vi "Update Parameter Value.vi"(8 "error in (no error)":errorcluster, 9 "Value":dbl format="%#_13g", 10 "Parameter":string, 11 "Async Message in":refnum<class "Async Message.lvclass">) -> (0 "error out":errorcluster, 3 "Async Message out":refnum<class "Async Message.lvclass">)   [LabVIEW 2020, in "BCI-1553 API.lvlib" / "Async Message.lvclass"]
doc: "This method allows a parameter value stored in an Asynchronous Message to be updated."
uses:
  Async Message.lvclass
  Async Message.lvclass/Async Message.ctl
  BCI-1553 API.lvlib
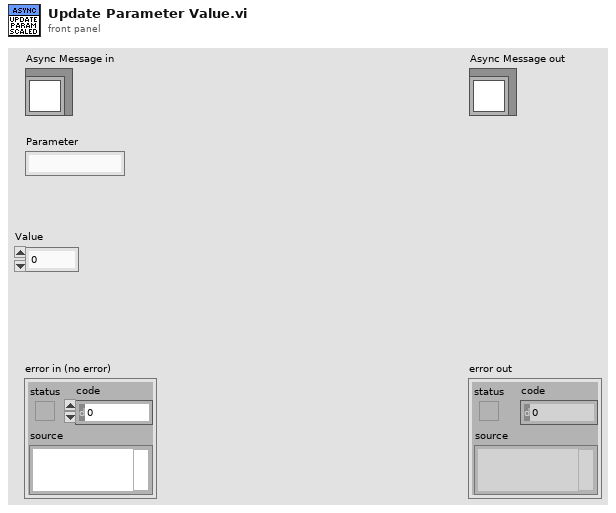
[diagram p1: front panel]
types:
  T1 = typedef "BCI-1553 API.lvlib/Parameter Table Data.ctl" = cluster{"Parameter Name":string, "Base Word":u16, "Address":u16, "Value":u64, "Mask":u16[], "Scaling Info":T2}
  T2 = typedef "BCI-1553 API.lvlib/Scaling Information.ctl" = cluster{"Bit Offset":i32, "Bit Count":i32, "LSB Resolution":dbl, "2's Complement":bool, "Big Endian":bool, "Sign Bit":bool}
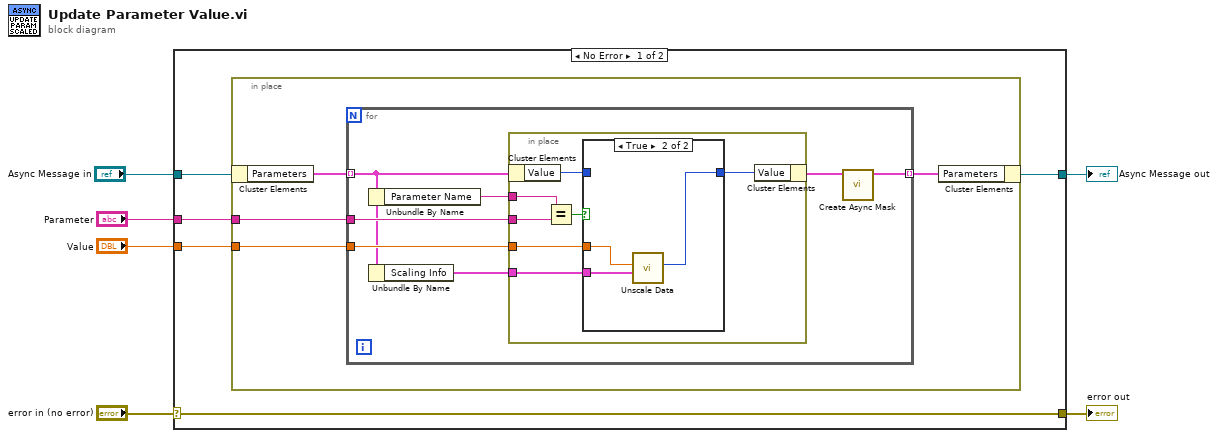
[diagram p0: block diagram]
diagram:
  n1 = case shown="No Error" "error in (no error)" {
    selector: "error in (no error)" -> [w11 w35]
    tunnel: [w11 w35] -> w5
    tunnel: [w7 w34] -> w3
    tunnel: "Async Message in" -> [w8 w34]
    tunnel: "Parameter" -> [w10 _]
    tunnel: "Value" -> [w9 _]
    frame No Error {
      n2 = in-place {
        in-place-border: w10 -> [w15]
        in-place-border: w9 -> [w14]
        n3 = in-place-cluster #1(w8) -> ("Parameters"=w13:T1[])
        n4 = for {
          tunnel: w13 -> [w20] mode=indexing
          tunnel: w15 -> [w22]
          tunnel: w14 -> [w21]
          tunnel: [w16] -> w12 mode=indexing
          n5 = Unbundle By Name(w20) -> ("Parameter Name"=w18:string)
          n6 = Unbundle By Name(w20) -> ("Scaling Info"=w19:T2)
          n7 = in-place {
            in-place-border: w22 -> [w29]
            in-place-border: w21 -> [w25]
            in-place-border: w19 -> [w24]
            in-place-border: w18 -> [w23]
            n8 = in-place-cluster #2(w20) -> ("Value"=w27:u64)
            n9 = Equal?(x=w23, y=w29) -> (x = y?=w28:bool)
            n10 = case shown="True" w28 {
              tunnel: w27 -> [w30 _]
              tunnel: [w30 w31] -> w26
              tunnel: w25 -> [_ w33]
              tunnel: w24 -> [_ w32]
              frame False {
              }
              frame True {
                n11 = call "Unscale Data.vi"("Scaling Info"=w32, "Scaled Value"=w33) -> ("Raw Value"=w31:u64)  [unwired: 8 in, 1 out]
              }
            }
            n12 = in-place-cluster #2("Value"=w26) -> (w17:T1)
          }
          n13 = call "Create Async Mask.vi"("Parameter In"=w17) -> ("Parameter Out"=w16:T1)  [unwired: 9 in, 1 out]
        }
        n14 = in-place-cluster #1("Parameters"=w12) -> (w7:refnum<class "Async Message.lvclass">)
      }
    }
    frame Error {
    }
  }
  "error out" <- w5
  "Async Message out" <- w3
